vi "set_prefix.vi"(8 "error in (no error)":errorcluster, 10 "_prefix_":string, 11 "self in":refnum<class "Identifier.lvclass">) -> (0 "error out":errorcluster, 3 "self out":refnum<class "Identifier.lvclass">)   [LabVIEW 2020, in "mlir.lvlib" / "Identifier.lvclass"]
uses:
  Identifier.lvclass
  Identifier.lvclass/Identifier.ctl
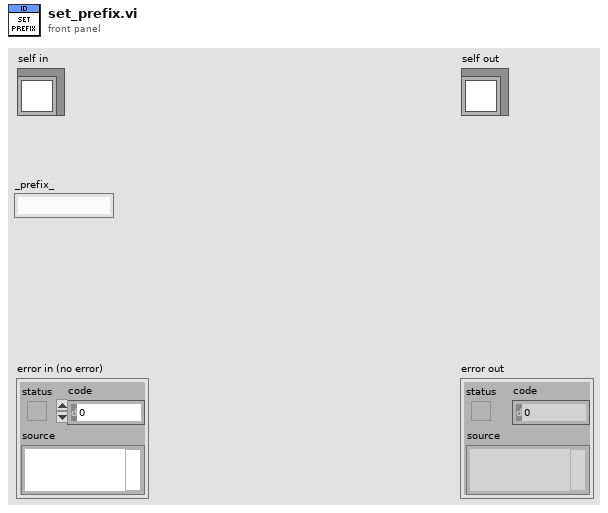
[diagram p1: front panel]
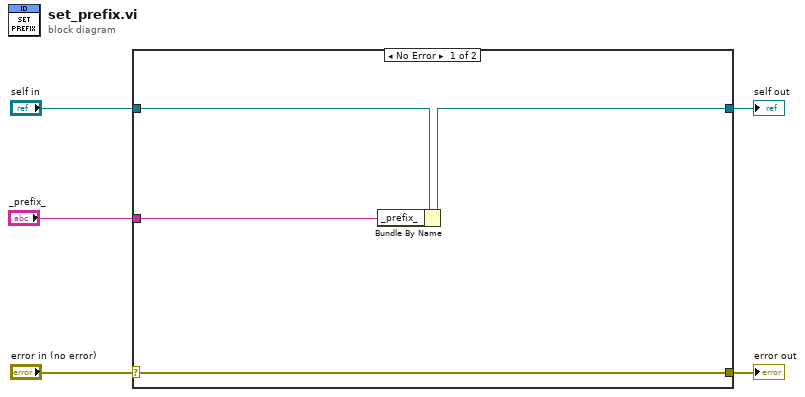
[diagram p0: block diagram]
diagram:
  n1 = case shown="No Error" "error in (no error)" {
    selector: "error in (no error)" -> [w6 w11]
    tunnel: [w6 w11] -> w4
    tunnel: [w8 w10] -> w2
    tunnel: "self in" -> [w9 w10]
    tunnel: "_prefix_" -> [w7 _]
    frame No Error {
      n2 = Bundle By Name(cluster=w9, "_prefix_"=w7) -> (w8:refnum<class "Identifier.lvclass">)
    }
    frame Error {
    }
  }
  "error out" <- w4
  "self out" <- w2
